vi "QPSK Modulation.vi"(10 "pulse shaping filter (none)":T1(ring), 11 "coerced IQ rate":dbl) -> (2 "output complex waveform":T2 {"Y" format="%.3f"; "dt" format="%^.2e"; "t0" format="%.4f"}, 3 "output bit stream":i8[](array[numeric]))   [LabVIEW 2026]
uses:
  <vilib>/addons/Modulation/Analog/controls/Complex Data Waveform.ctl
  <vilib>/addons/Modulation/Analog/support/mod_Set Error Source.vi
  <vilib>/addons/Modulation/Analog/support/Validators/mod_Fractional Resample Validate.vi
  <vilib>/addons/Modulation/Analog/support/Validators/mod_Check Flush State.vi
  <vilib>/addons/Modulation/Analog/support/mod_FractionalResampler.vi
  <vilib>/addons/Modulation/Analog/support/mod_Integer Rate Interpolation.vi
  <vilib>/addons/Modulation/Analog/support/Validators/mod_Validate Complex Waveform.vi
  <vilib>/addons/Modulation/Analog/support/mod_PerformResampling.vi
  <vilib>/addons/Modulation/Analog/support/Validators/mod_WFErrorHandler.vi
  <vilib>/addons/Modulation/Digital/General/MT Generate PSK System Parameters(M).vi
  <vilib>/addons/Modulation/Digital/Support/Common/Validators/mod_Generate Filter Coefficients Validate.vi
  <vilib>/addons/Modulation/Digital/General/subVIs/mod_Generate Filter Coefficients.vi
  <vilib>/Utility/error.llb/Error Cluster From Error Code.vi
  <vilib>/addons/Modulation/Analog/support/mod_Resampling Factors.vi
  <vilib>/addons/Modulation/Analog/support/mod_ResamplingFilter.vi
  <vilib>/addons/Modulation/Analog/support/mod_Generate Integer Interpolation Filter.vi
  <vilib>/addons/Modulation/niAMT.lvlib
  <vilib>/addons/Modulation/niDMT.lvlib
panel:
  out "symbols out":cdb[](array[numeric]) format="%.2f"
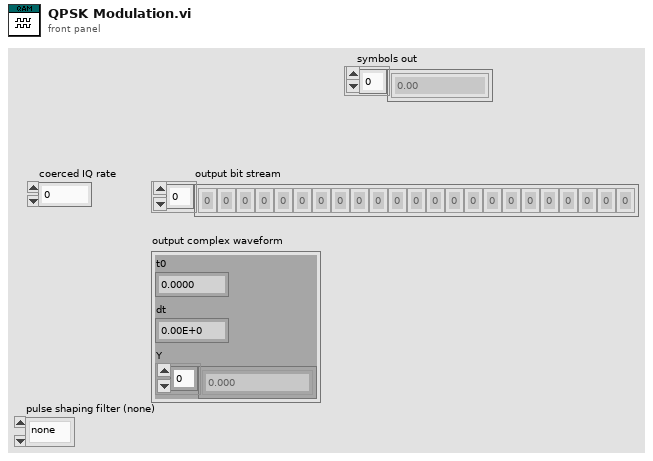
[diagram p1: front panel]
types:
  T1 = enum16{"none", "Raised Cosine", "Root Raised Cos", "Gaussian"}
  T2 = typedef "niAMT.lvlib/Complex Data Waveform.ctl" = cluster{"t0":dbl, "dt":dbl, "Y":cdb[]}
  T3 = enum16{"FSK", "PSK", "QAM", "MSK", "PAM", "ASK", "CPM"}
  T4 = cluster{"samples per symbol (16)":i32, "symbol map":cdb[], "differential PSK":enum16{"disable", "enable"}, "PSK type":u16}
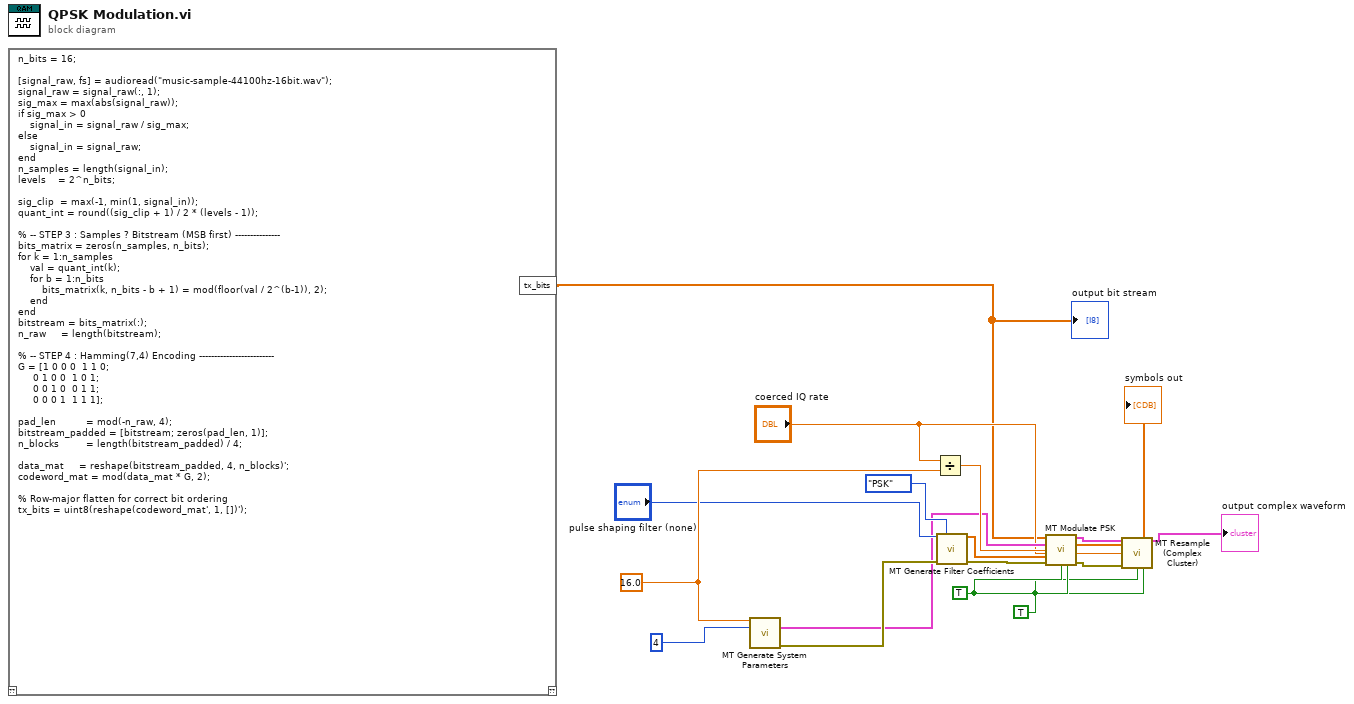
[diagram p0: block diagram]
diagram:
  w16 = TRUE ("reset? (T)")
  w17 = 16.0 ("y")
  w8 = TRUE ("reset? (T)")
  n1 = script code="n_bits = 16;\n\n[signal_raw, fs] = audioread(\"music-sample-44100hz-16bit.wav\");\nsignal_raw = signal_raw(:, 1);\nsig_max = max(abs(signal_raw));\nif sig_max > 0\n    signal_in = signal_raw / sig_max;\nelse\n    signal_in = signal_raw;\nend\nn_samples = length(signal_in);\nlevels    = 2^n_bits;\n\nsig_clip  = max(-1, min(1, signal_in));\nquant_int = round((sig_clip + 1) / 2 * (levels - 1));\n\n% -- STEP 3 : Samples ? Bitstream (MSB first) ---------------\nbits_matrix = zeros(n_samples, n_bits);\nfor k = 1:n_samples\n    val = quant_int(k);\n    for b = 1:n_bits\n        bits_matrix(k, n_bits - b + 1) = mod(floor(val / 2^(b-1)), 2);\n    end\nend\nbitstream = bits_matrix(:);\nn_raw     = length(bitstream);\n\n% -- STEP 4 : Hamming(7,4) Encoding -------------------------\nG = [1 0 0 0  1 1 0;\n     0 1 0 0  1 0 1;\n     0 0 1 0  0 1 1;\n     0 0 0 1  1 1 1];\n\npad_len          = mod(-n_raw, 4);\nbitstream_padded = [bitstream; zeros(pad_len, 1)];\nn_blocks         = length(bitstream_padded) / 4;\n\ndata_mat     = reshape(bitstream_padded, 4, n_blocks)';\ncodeword_mat = mod(data_mat * G, 2);\n\n% Row-major flatten for correct bit ordering\ntx_bits = uint8(reshape(codeword_mat', 1, [])');"() -> ("tx_bits"=w1:dbl[])  [unwired: 1 in, 1 out]
  "output bit stream" <- w1
  n2 = call-poly <vilib>:"MT Generate System Parameters.vi"("samples per symbol (16)"=w17, "M-PSK (4)"=4) -> ("PSK system parameters"=w10:T4, "error out"=w13:errorcluster)  [unwired: 11 in, 1 out]
  n3 = Divide(x="coerced IQ rate", y=w17) -> (x/y=w14:dbl)
  n4 = call <vilib>:"MT Generate Filter Coefficients.vi"("pulse shaping filter (none)"="pulse shaping filter (none)", "modulation type"=T3."PSK", "error in (no error)"=w13) -> ("pulse shaping filter coefficients"=w9:dbl[], "error out"=w12:errorcluster)  [unwired: 10 in, 1 out]
  n5 = call <vilib>:"MT Modulate PSK.vi"("input bit stream"=w1, "PSK system parameters"=w10, "symbol rate (Hz)"=w14, "pulse shaping filter coefficients"=w9, "error in (no error)"=w12, "reset? (T)"=w16, "flush buffers? (F)"=w16) -> ("output complex waveform"=w6:T2, "symbols out"=→"symbols out":cdb[], "error out"=w7:errorcluster)  [unwired: 6 in]
  n6 = call <vilib>:"MT Resample (Complex Cluster).vi"("input complex waveform"=w6, "desired sample rate (Hz)"="coerced IQ rate", "error in (no error)"=w7, "reset? (T)"=w8, "flush buffers? (F)"=w8) -> ("output complex waveform"=→"output complex waveform":T2)  [unwired: 9 in, 1 out]
